vi "Obis Engine.vi"(0 "Obis Notifier":string="Not a Name", 11 "COM Port":string[](array[string])) -> ()   [LabVIEW 2016]
uses:
  Laser Controls/Laser Status.ctl
  Laser Controls/Laser Notifier Element.ctl
  Laser Controls/Laser Actions.ctl
  Laser Controls/Laser Settings.ctl
  Laser Controls/Laser Parameters.ctl
  <vilib>/Instr/_visa.llb/VISA Configure Serial Port (Instr).vi
panel:
  out "Startup Error":errorcluster
  in  "Get Power":bool
  out "Status":T1
  out "Light Emission?":bool
  out "Enabled (Interlock)?":bool
  in  "Get Status":bool
  in  "Laser Power (mW)":dbl
  in  "Laser On/Off":bool
  in  "Quit":bool
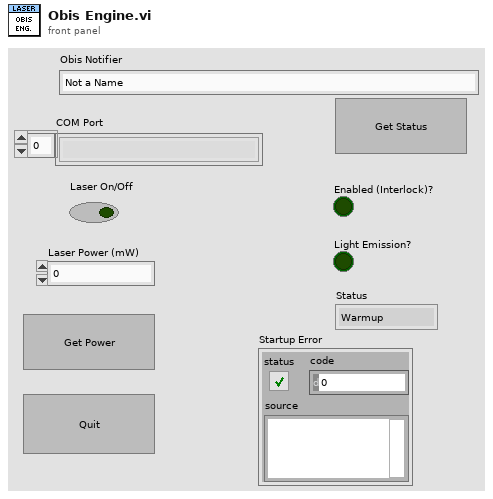
[diagram p1: front panel]
types:
  T1 = typedef "Laser Status.ctl" = enum16{"Warmup", "Ready", "Emission", "Tuning", "Error"}
  T2 = typedef "Laser Notifier Element.ctl" = cluster{"Laser Action":T3, "Received?":bool, "Enabled (Interlock)?":bool, "Light Emission?":bool, "Power (mW)":dbl, "Settings":T4, "Status":T1, "Error":errorcluster}
  T3 = typedef "Laser Actions.ctl" = enum16{"Error Check", "Set On/Off", "Set Power", "Set Parameter", "Get Power", "Get Status", "Get Parameter", "Quit"}
  T4 = typedef "Laser Settings.ctl" = cluster{"Laser Parameters":T5, "Value":dbl}
  T5 = typedef "Laser Parameters.ctl" = enum16{"Wavelength (nm)", "Pulsing?", "Rep. Rate"}
  T6 = enum32{"Invalid", "Standard", "Closed", "Hidden", "Minimized", "Maximized"}
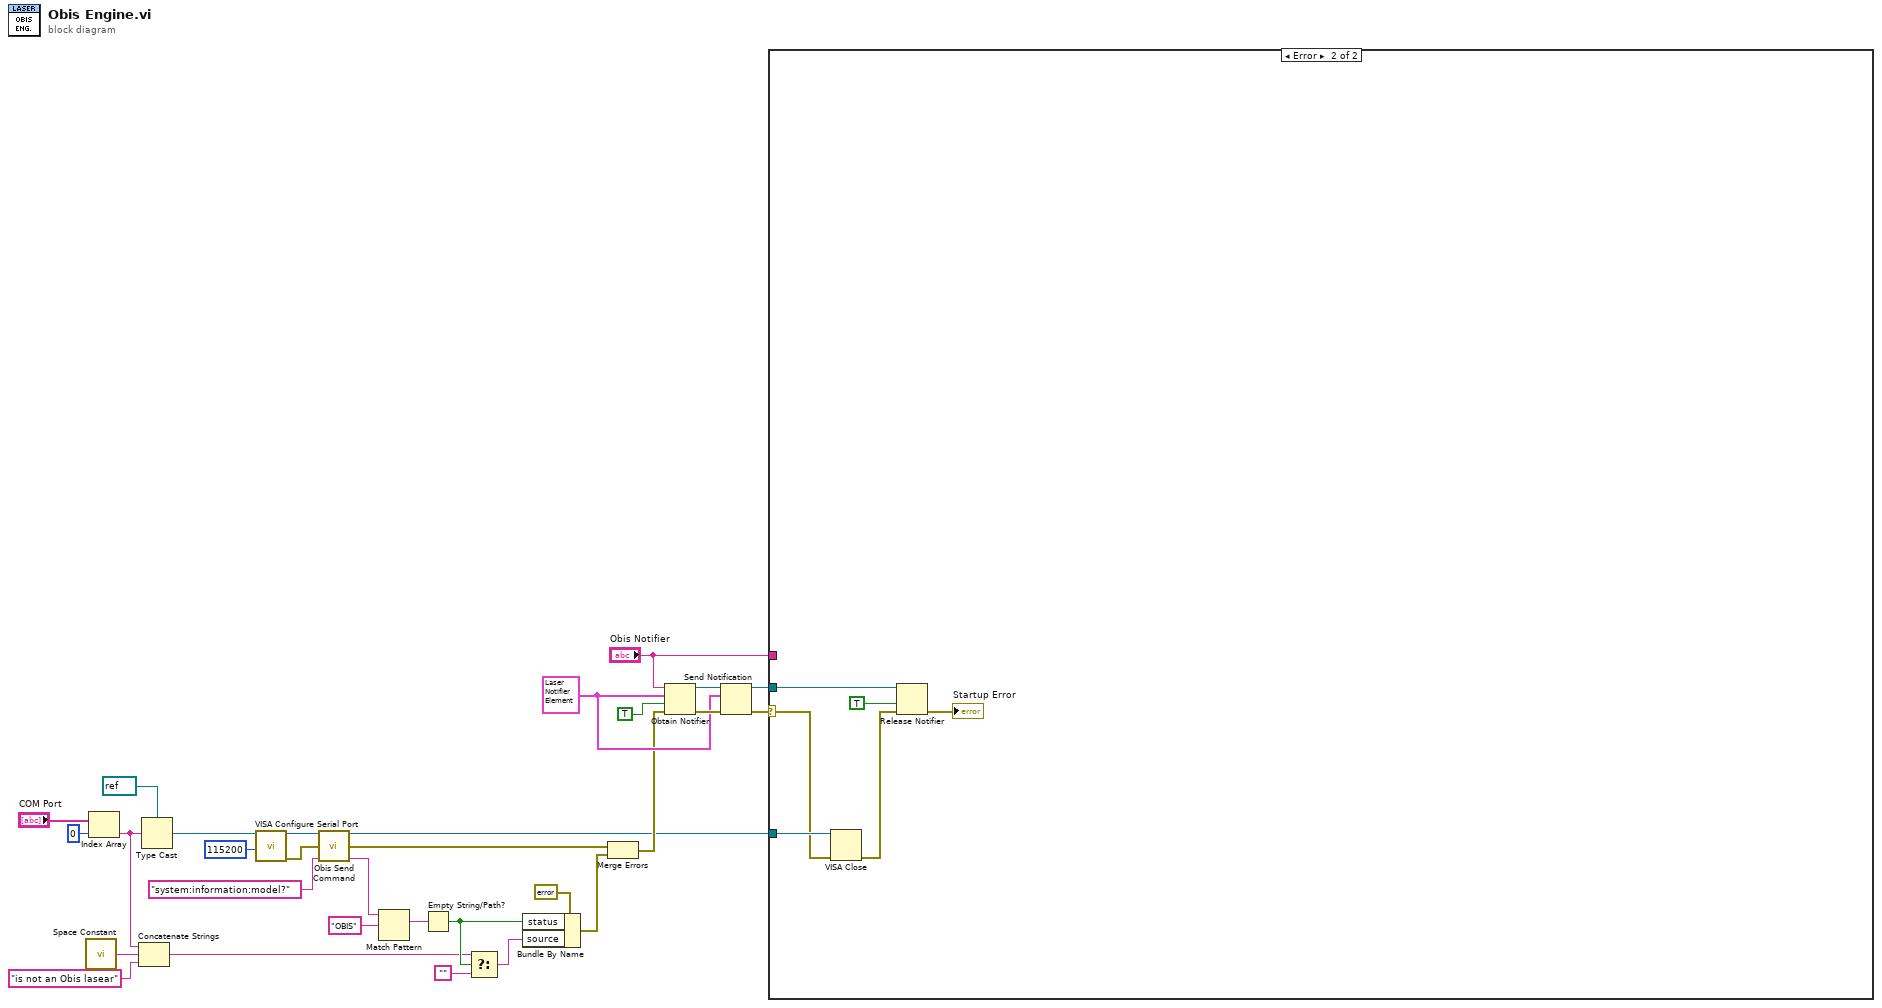
[diagram p0: block diagram]
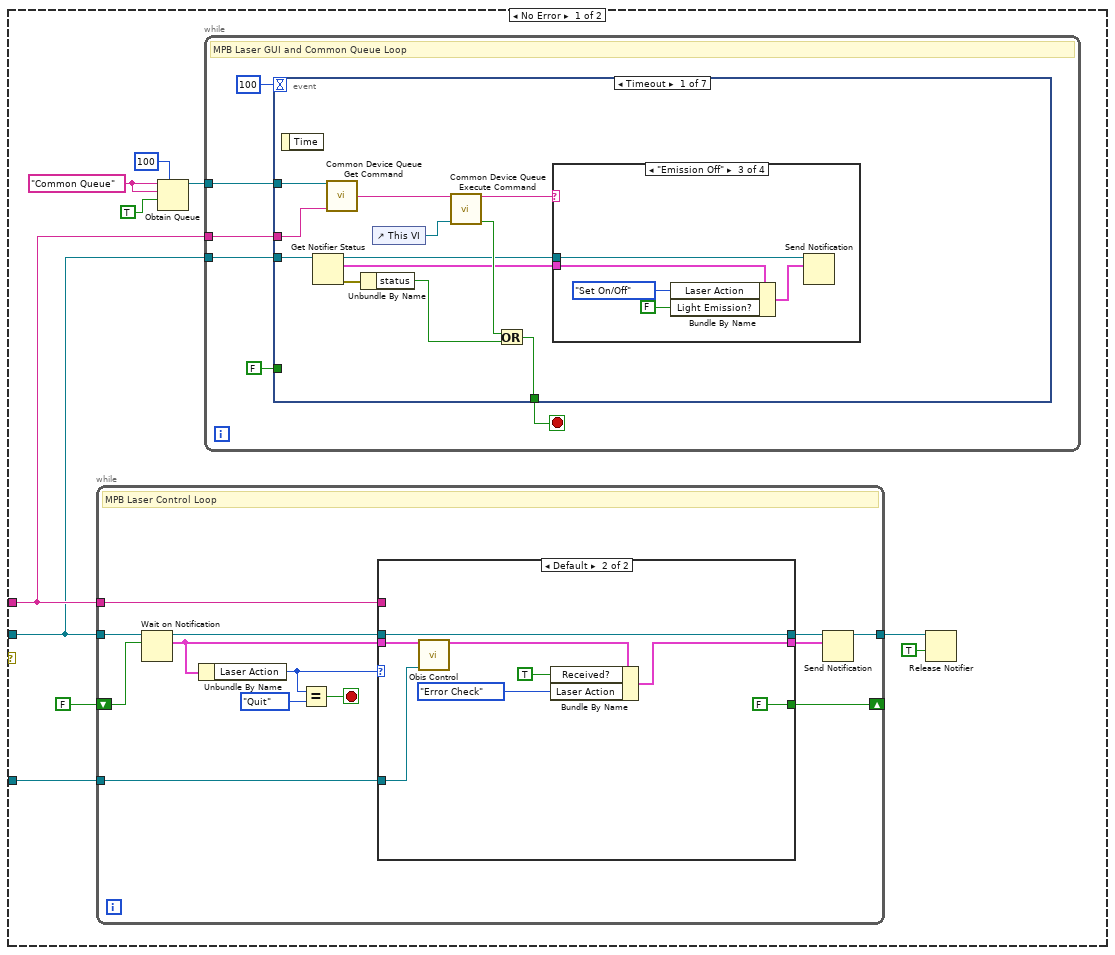
[diagram p2: hidden frame]
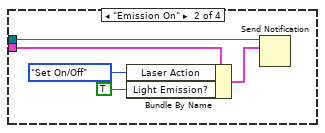
[diagram p4: hidden frame]
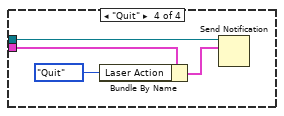
[diagram p5: hidden frame]
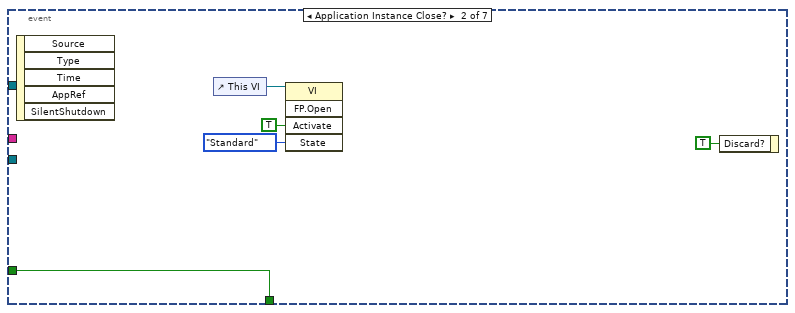
[diagram p6: hidden frame]
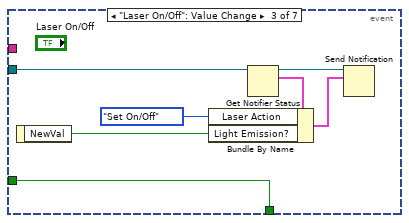
[diagram p7: hidden frame]
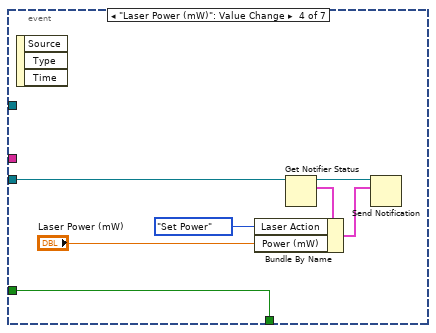
[diagram p8: hidden frame]
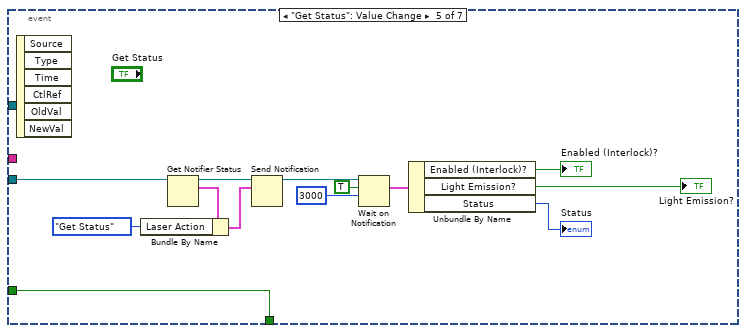
[diagram p9: hidden frame]
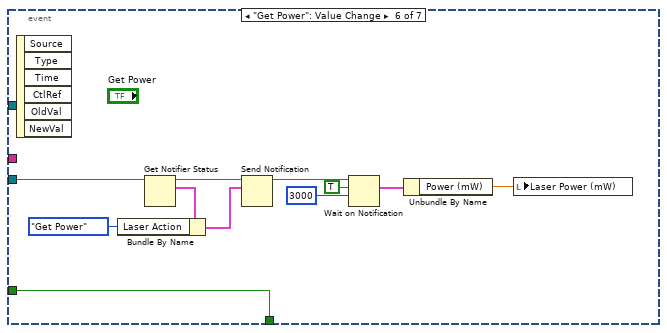
[diagram p10: hidden frame]
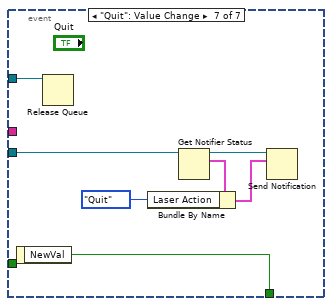
[diagram p11: hidden frame]
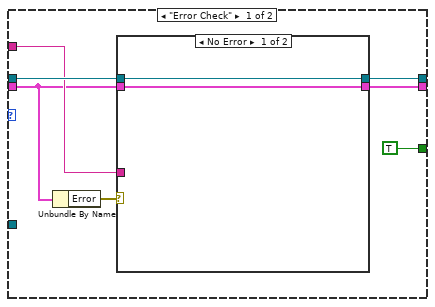
[diagram p12: hidden frame]
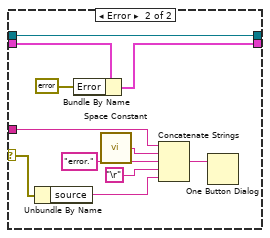
[diagram p13: hidden frame]
diagram:
  w21 = T2 {"Laser Action"=enum."Get Status", "Received?"=FALSE, "Enabled (Interlock)?"=FALSE, "Light Emission?"=FALSE, "Power (mW)"=0.0, "Settings"={"Laser Parameters"=enum."Wavelength (nm)", "Value"=0.0}, "Status"=enum."Error", "Error"={"status"=FALSE, "code"=0, "source"=""}} ("Laser Notifier Element")
  n1 = call <vilib>:"Space Constant.vi"() -> ("String"=w12:string)
  n2 = Index Array(array="COM Port", index=0) -> (element=w13:string)
  n3 = Concatenate Strings(w13, w12, "is not an Obis lasear" ("string")) -> (w9:string)
  n4 = Type Cast(type=refnum<visa-resource-name> refnum ("VISA resource name"), x=w13) -> (*(type *) &x=w3:refnum<visa-resource-name>)
  n5 = call-poly "VISA Configure Serial Port"("VISA resource name"=w3, "baud rate (9600)"=u32 115200) -> ("VISA resource name out"=w2:refnum<visa-resource-name>, "error out"=w1:errorcluster)  [unwired: 12 in]
  n6 = call "Obis Send Command.vi"("VISA Ref"=w2, "Error In"=w1, "Command"="system:information:model?") -> ("VISA Ref Out"=w16:refnum<visa-resource-name>, "Error Out"=w18:errorcluster, "Response"=w20:string)  [unwired: 10 in]
  n7 = Match Pattern(string=w20, regular expression="OBIS") -> (match substring=w15:string)  [unwired: 1 in, 3 out]
  n8 = Empty String/Path?(string/path=w15) -> (empty?=w10:bool)
  n9 = Select(t=w9, s=w10, f="") -> (s? t:f=w8:string)
  n10 = Bundle By Name(cluster=errorcluster {"status"=FALSE, "code"=0, "source"=""} ("error in"), "status"=w10, "source"=w8) -> (w6:errorcluster)
  n11 = Merge Errors(w18, w6) -> (w17:errorcluster)
  n12 = Obtain Notifier(name (unnamed)="Obis Notifier", notification data type=w21, create if not found? (T)=TRUE, error in (no error)=w17) -> (notifier out=w29:refnum<notifier>, error out=w28:errorcluster)  [unwired: 1 out]
  n13 = Send Notification(notification=w21, notifier=w29, error in (no error)=w28) -> (notifier out=w27:refnum<notifier>, error out=w26:errorcluster)
  n14 = case shown="Error" w26 {
    selector: w26 -> [_ w165]
    tunnel: w27 -> [w32 w167]
    tunnel: "Obis Notifier" -> [w33 _]
    tunnel: w16 -> [w31 w166]
    frame No Error {
      w37 = "Common Queue" ("Unique Notifier Name")
      n15 = while {
        tunnel: w32 -> [w133]
        tunnel: [w134] -> w39
        shift-right: [w126] -> _
        shift-left: FALSE -> [w128]
        tunnel: w33 -> [w125]
        tunnel: w31 -> [w123]
        stop <- w135 stop-if-true
        # "MPB Laser Control Loop"
        n16 = Wait on Notification(notifier=w133, ignore previous (F)=w128) -> (notifier out=w132:refnum<notifier>, notification=w131:T2)  [unwired: 2 in, 2 out]
        n17 = Unbundle By Name(w131) -> ("Laser Action"=w130:T3)
        n18 = Equal?(x=w130, y=Laser_Actions."Quit") -> (x = y?=w135:bool)
        n19 = case shown="Default" w130 {
          tunnel: w132 -> [w142 w156]
          tunnel: [w141 w156] -> w129
          tunnel: w131 -> [w138 w158]
          tunnel: w125 -> [w140 _]
          tunnel: [w139 w162] -> w127
          tunnel: [TRUE FALSE] -> w126
          tunnel: w123 -> [_ w163]
          frame "Error Check" {
            n20 = Unbundle By Name(w138) -> ("Error"=w137:errorcluster)
            n21 = case shown="No Error" w137 {
              selector: w137 -> [_ w148]
              tunnel: w138 -> [w143 w152]
              tunnel: [w144 w150] -> w141
              tunnel: w142 -> [w144 w150]
              tunnel: w140 -> [_ w147]
              tunnel: [w143 w149] -> w139
              frame No Error {
              }
              frame Error {
                n22 = Unbundle By Name(w148) -> ("source"=w146:string)
                n23 = Bundle By Name(cluster=w152, "Error"=errorcluster {"status"=FALSE, "code"=0, "source"=""}) -> (w149:T2)
                n24 = call <vilib>:"Space Constant.vi"() -> ("String"=w155:string)
                n25 = Concatenate Strings(w147, w155, "error." ("string"), "\r", w146) -> (w153:string)
                n26 = One Button Dialog(message=w153) -> ()  [unwired: 1 in, 1 out]
              }
            }
          }
          frame Default {
            n27 = call "Obis Control.vi"("Laser Notifier Element"=w158, "VISA Ref"=w163) -> ("Laser Notifier Element"=w157:T2)  [unwired: 13 in]
            n28 = Bundle By Name(cluster=w157, "Received?"=TRUE, "Laser Action"=Laser_Actions."Error Check") -> (w162:T2)
          }
        }
        n29 = Send Notification(notification=w127, notifier=w129) -> (notifier out=w134:refnum<notifier>)  [unwired: 1 in, 1 out]
      }
      n30 = Obtain Queue(max queue size (-1, unlimited)=100, name (unnamed)=w37, element data type=w37, create if not found? (T)=TRUE) -> (queue out=w34:refnum<queue>)  [unwired: 1 in, 2 out]
      n31 = while {
        tunnel: w34 -> [w45]
        tunnel: w33 -> [w43]
        tunnel: w32 -> [w44]
        stop <- w42 stop-if-true
        # "MPB Laser GUI and Common Queue Loop"
        n32 = event shown="[0] Timeout" {
          selector: _ -> [_ _ _ _ _ _ _]
          dyn-events: _ -> [_ _ _ _ _ _ _]
          timeout: 100 -> [_ _ _ _ _ _ _]
          tunnel: w45 -> [w52 _ _ _ _ _ w122]
          tunnel: w44 -> [w51 _ w79 w86 w100 w111 w121]
          tunnel: w43 -> [w50 _ _ _ _ _ _]
          tunnel: [w49 w77 w84 w91 w104 w115 w119] -> w42
          tunnel: FALSE -> [_ w77 w84 w91 w104 w115 _]
          event Timeout {
            n33 = event-data() -> ()  [unwired: 1 in, 1 out]
            n34 = Get Notifier Status(notifier=w51) -> (notifier out=w53:refnum<notifier>, current notification=w48:T2, error out=w58:errorcluster)  [unwired: 1 in, 2 out]
            n35 = call "Common Device Queue Get Command.vi"("Common Queue"=w52, "Notifier Name"=w50) -> ("Command"=w57:string)  [unwired: 12 in, 1 out]
            n36 = Unbundle By Name(w58) -> ("status"=w55:bool)
            n37 = control-ref of="This VI"() -> (w56:refnum<vi>)
            n38 = call "Common Device Queue Execute Command.vi"("Common Command"=w57, "VI Refnum"=w56) -> ("Common Command"=w47:string, "Quit?"=w54:bool)  [unwired: 12 in]
            n39 = Or(x=w54, y=w55) -> (x .or. y?=w49:bool)
            n40 = case shown="\"Emission Off\"" w47 {
              tunnel: w53 -> [_ w63 w68 w72]
              tunnel: w48 -> [_ w62 w67 w71]
              frame Default {
              }
              frame "Emission On" {
                n41 = Bundle By Name(cluster=w62, "Laser Action"=Laser_Actions."Set On/Off", "Light Emission?"=TRUE) -> (w61:T2)
                n42 = Send Notification(notification=w61, notifier=w63) -> ()  [unwired: 1 in, 2 out]
              }
              frame "Emission Off" {
                n43 = Bundle By Name(cluster=w67, "Laser Action"=Laser_Actions."Set On/Off", "Light Emission?"=FALSE) -> (w66:T2)
                n44 = Send Notification(notification=w66, notifier=w68) -> ()  [unwired: 1 in, 2 out]
              }
              frame "Quit" {
                n45 = Bundle By Name(cluster=w71, "Laser Action"=Laser_Actions."Quit") -> (w70:T2)
                n46 = Send Notification(notification=w70, notifier=w72) -> ()  [unwired: 1 in, 2 out]
              }
            }
          }
          event Application Instance Close? {
            n47 = event-data() -> ()  [unwired: 1 in, 5 out]
            n48 = control-ref of="This VI"() -> (w74:refnum<vi>)
            n49 = invoke class="VI" method="FP.Open"(reference=w74, "Activate"=TRUE ("Activate?"), "State"=T6."Standard") -> ()  [unwired: 2 in, 5 out]
            n50 = event-data("Discard?"=TRUE) -> ()  [unwired: 1 in, 1 out]
          }
          event "Laser On/Off": Value Change {
            n51 = event-data() -> ("NewVal"=w78:bool)  [unwired: 1 in]
            n52 = Get Notifier Status(notifier=w79) -> (notifier out=w83:refnum<notifier>, current notification=w82:T2)  [unwired: 1 in, 3 out]
            n53 = Bundle By Name(cluster=w82, "Laser Action"=Laser_Actions."Set On/Off", "Light Emission?"=w78) -> (w80:T2)
            n54 = Send Notification(notification=w80, notifier=w83) -> ()  [unwired: 1 in, 2 out]
          }
          event "Laser Power (mW)": Value Change {
            n55 = event-data() -> ()  [unwired: 1 in, 3 out]
            n56 = Get Notifier Status(notifier=w86) -> (notifier out=w90:refnum<notifier>, current notification=w89:T2)  [unwired: 1 in, 3 out]
            n57 = Bundle By Name(cluster=w89, "Laser Action"=Laser_Actions."Set Power", "Power (mW)"="Laser Power (mW)") -> (w87:T2)
            n58 = Send Notification(notification=w87, notifier=w90) -> ()  [unwired: 1 in, 2 out]
          }
          event "Get Status": Value Change {
            n59 = event-data() -> ()  [unwired: 1 in, 6 out]
            n60 = Get Notifier Status(notifier=w100) -> (notifier out=w103:refnum<notifier>, current notification=w102:T2)  [unwired: 1 in, 3 out]
            n61 = Bundle By Name(cluster=w102, "Laser Action"=Laser_Actions."Get Status") -> (w101:T2)
            n62 = Send Notification(notification=w101, notifier=w103) -> (notifier out=w99:refnum<notifier>)  [unwired: 1 in, 1 out]
            n63 = Wait on Notification(notifier=w99, ignore previous (F)=TRUE, timeout in ms (-1)=3000) -> (notification=w96:T2)  [unwired: 1 in, 3 out]
            n64 = Unbundle By Name(w96) -> ("Enabled (Interlock)?"=→"Enabled (Interlock)?":bool, "Light Emission?"=→"Light Emission?":bool, "Status"=→"Status":T1)
          }
          event "Get Power": Value Change {
            n65 = event-data() -> ()  [unwired: 1 in, 6 out]
            n66 = Get Notifier Status(notifier=w111) -> (notifier out=w114:refnum<notifier>, current notification=w113:T2)  [unwired: 1 in, 3 out]
            n67 = Bundle By Name(cluster=w113, "Laser Action"=Laser_Actions."Get Power") -> (w112:T2)
            n68 = Send Notification(notification=w112, notifier=w114) -> (notifier out=w110:refnum<notifier>)  [unwired: 1 in, 1 out]
            n69 = Wait on Notification(notifier=w110, ignore previous (F)=TRUE, timeout in ms (-1)=3000) -> (notification=w107:T2)  [unwired: 1 in, 3 out]
            n70 = Unbundle By Name(w107) -> ("Power (mW)"=w106:dbl)
            n71 = local write "Laser Power (mW)"(w106) -> ()
          }
          event "Quit": Value Change {
            n72 = event-data() -> ("NewVal"=w119:bool)  [unwired: 1 in]
            n73 = Release Queue(queue=w122) -> ()  [unwired: 2 in, 3 out]
            n74 = Get Notifier Status(notifier=w121) -> (notifier out=w120:refnum<notifier>, current notification=w118:T2)  [unwired: 1 in, 3 out]
            n75 = Bundle By Name(cluster=w118, "Laser Action"=Laser_Actions."Quit") -> (w116:T2)
            n76 = Send Notification(notification=w116, notifier=w120) -> ()  [unwired: 1 in, 2 out]
          }
        }
      }
      n77 = Release Notifier(notifier=w39, force destroy? (F)=TRUE) -> ()  [unwired: 1 in, 3 out]
    }
    frame Error {
      n78 = VISA Close(VISA resource name=w166, error in (no error)=w165) -> (error out=w168:errorcluster)
      n79 = Release Notifier(notifier=w167, force destroy? (F)=TRUE, error in (no error)=w168) -> (error out=→"Startup Error":errorcluster)  [unwired: 2 out]
    }
  }
